vi "Create Error Qs.vi"(0 "Number of Error Queues to Create":i32, 11 "error in (no error)":errorcluster) -> (4 "Error Queues":refnum<queue>[](array[refnum]), 6 "Error Publishing Queue":refnum<queue>, 15 "error out":errorcluster)   [LabVIEW 2013, in "AIT 664 Custom Device.lvlib"]
uses:
  AIT 664 Custom Device.lvlib
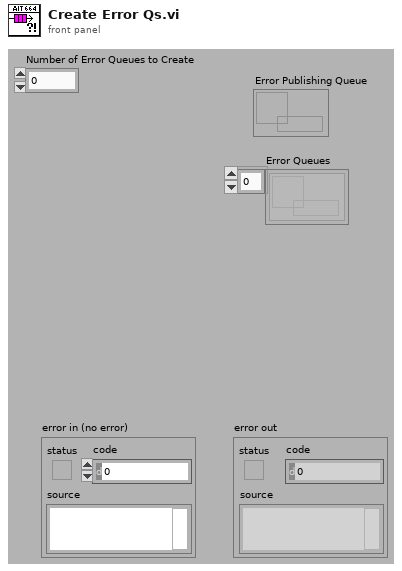
[diagram p1: front panel]
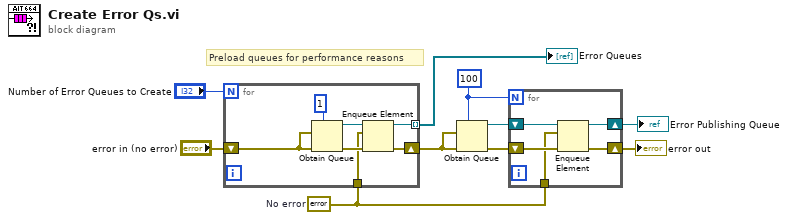
[diagram p0: block diagram]
diagram:
  w3 = errorcluster {"status"=FALSE, "code"=0, "source"=""}  # No error
  w2 = 100 ("max queue size (-1, unlimited)")
  # "Preload queues for performance reasons"
  n1 = for {
    N: "Number of Error Queues to Create" -> [_]
    shift-right: [w13] -> w8
    shift-left: "error in (no error)" -> [w17]
    tunnel: [w14] -> w9 mode=indexing
    tunnel: w3 -> [w11]
    n2 = Obtain Queue(max queue size (-1, unlimited)=1, element data type=w17, error in (no error)=w17) -> (queue out=w15:refnum<queue>, error out=w12:errorcluster)  [unwired: 2 in, 1 out]
    n3 = Enqueue Element(queue=w15, element=w11, error in (no error)=w12) -> (queue out=w14:refnum<queue>, error out=w13:errorcluster)  [unwired: 1 in, 1 out]
  }
  "Error Queues" <- w9
  n4 = Obtain Queue(max queue size (-1, unlimited)=w2, element data type=w8, error in (no error)=w8) -> (queue out=w6:refnum<queue>, error out=w7:errorcluster)  [unwired: 2 in, 1 out]
  n5 = for {
    N: w2 -> [_]
    shift-right: [w19] -> w4
    shift-left: w7 -> [w22]
    shift-right: [w20] -> w5
    shift-left: w6 -> [w21]
    tunnel: w3 -> [w18]
    n6 = Enqueue Element(queue=w21, element=w18, error in (no error)=w22) -> (queue out=w20:refnum<queue>, error out=w19:errorcluster)  [unwired: 1 in, 1 out]
  }
  "error out" <- w4
  "Error Publishing Queue" <- w5
